vi "Popuplate diagnostics selecction.vi"(8 "error in (no error)":errorcluster, 10 "MainDiagnostics":refnum<vi>, 11 "Diagnostics in":T1) -> (0 "error out":errorcluster)   [LabVIEW 2019, in "ZenGage v3.0 UI.lvclass"]
uses:
  ZenGage v3.0 UI.lvclass
  Type Definitions/Diagnostics/Diagnostics(Cluster).ctl
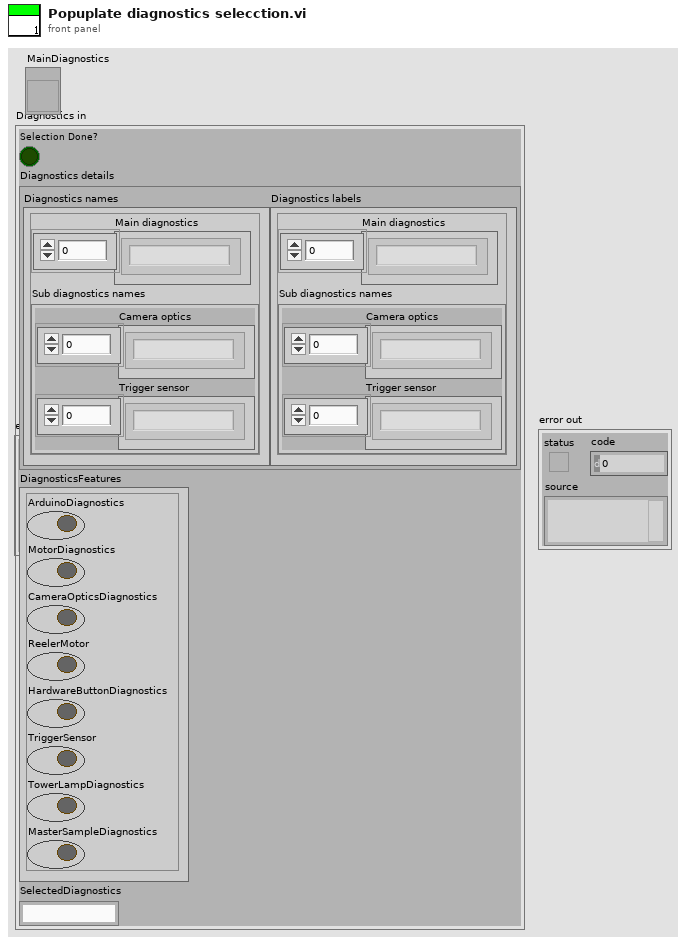
[diagram p1: front panel]
types:
  T1 = typedef "ZenGage v3.0 UI.lvclass/Diagnostics(Cluster).ctl" = cluster{"Selection Done?":bool, "Diagnostics details":cluster{"Diagnostics names":cluster{"Main diagnostics":string[], "Sub diagnostics names":cluster{"Camera optics":string[], "Trigger sensor":string[]}}, "Diagnostics labels":cluster{"Main diagnostics":string[], "Sub diagnostics names":cluster{"Camera optics":string[], "Trigger sensor":string[]}}}, "DiagnosticsFeatures":cluster{"ArduinoDiagnostics":bool, "MotorDiagnostics":bool, "CameraOpticsDiagnostics":bool, "ReelerMotor":bool, "HardwareButtonDiagnostics":bool, "TriggerSensor":bool, "TowerLampDiagnostics":bool, "MasterSampleDiagnostics":bool}, "SelectedDiagnostics":string}
  T2 = cluster{"ArduinoDiagnostics":bool, "MotorDiagnostics":bool, "CameraOpticsDiagnostics":bool, "ReelerMotor":bool, "HardwareButtonDiagnostics":bool, "TriggerSensor":bool, "TowerLampDiagnostics":bool, "MasterSampleDiagnostics":bool}
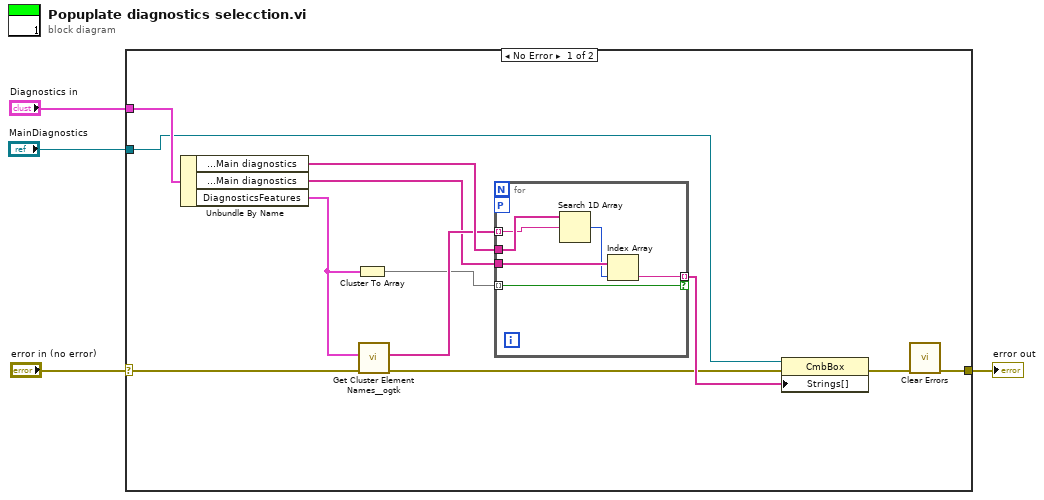
[diagram p0: block diagram]
diagram:
  n1 = case shown="No Error" "error in (no error)" {
    selector: "error in (no error)" -> [w8 w23]
    tunnel: [w7 w23] -> w3
    tunnel: "Diagnostics in" -> [w16 _]
    tunnel: "MainDiagnostics" -> [w6 _]
    frame No Error {
      n2 = Unbundle By Name(w16) -> ("Diagnostics details.Diagnostics names.Main diagnostics"=w15:string[], "Diagnostics details.Diagnostics labels.Main diagnostics"=w13:string[], "DiagnosticsFeatures"=w5:T2)
      n3 = Cluster To Array(cluster=w5) -> (array=w12:bool[])
      n4 = call <userlib>:"Get Cluster Element Names__ogtk.vi"("error in (no error)"=w8, "Cluster"=w5) -> ("error out"=w10:errorcluster, "Element Names"=w14:string[])  [unwired: 8 in]
      n5 = for {
        tunnel: w15 -> [w22]
        tunnel: w14 -> [w21] mode=indexing
        tunnel: w13 -> [w20]
        tunnel: w12 -> [w17] mode=indexing
        tunnel: [w18] -> w11 mode=indexing if=w17
        workers-P: _ -> [_]
        n6 = Search 1D Array(1D array=w22, element=w21) -> (index of element=w19:i32)  [unwired: 1 in]
        n7 = Index Array(array=w20, index=w19) -> (element=w18:string)
      }
      n8 = property class="CmbBox"(reference=w6, error in=w10, "Strings[]"=w11) -> (error out=w9:errorcluster)  [unwired: 1 out]
      n9 = call <vilib>:"Clear Errors.vi"("error in (no error)"=w9) -> ("error out"=w7:errorcluster)  [unwired: 5 in, 1 out]
    }
    frame Error {
    }
  }
  "error out" <- w3
